vi "OperateClick.vi"(3 "XRef":refnum<vi>, 4 "Point":T1, 5 "State In":T3={"Input Type"=variant(dbl 0.0), "Width"=0, "Typedef Name"="", "Value Type"=variant, "Selection"=0, "Options"=[], "Selections"=[], "Display Selections"=[], "Element Names"=[], "Typedef Name Width"=0, "Display Selection Width"=[], "Code Generated"=FALSE}) -> (0 "Reply":string[](array[string]), 2 "State Out":T3={"Input Type"=variant(dbl 0.0), "Width"=0, "Typedef Name"="", "Value Type"=variant, "Selection"=0, "Options"=[], "Selections"=[], "Display Selections"=[], "Element Names"=[], "Typedef Name Width"=0, "Display Selection Width"=[], "Code Generated"=FALSE})   [LabVIEW 2015, in "Read-Write-Signals.xnode"]
doc: "This ability VI is called when a user operate clicks on your XNode. Point is the point of the click relative to the top-left corner of your XNode. If you wish to show a menu in response to a user's operate click, issue the reply \"ShowMenu\". It is an error to issue this reply if you have not implemented the BuildMenu and SelectMenu ability VIs.\n\nDefault behavior: None.\n\nThis ability provides UI and OS messages are handled.\n\nSee also: BuildMenu3, SelectMenu3"
uses:
  Read-Write-Signals.xnode
  State.ctl
  Read-Write-Signals Item.ctl
  Read-Write-Signals Sub Item.ctl
  Read-Write-Signals Sub Item Type.ctl
  Read-Write-Signals Selection.ctl
  Read-Write-Signals Display Selection.ctl
  <vilib>/XNodeSupport/XNodePoint.ctl
  <vilib>/XNodeSupport/XNodeInt.ctl
  <vilib>/XNodeSupport/NI_XNodeSupport.lvlib
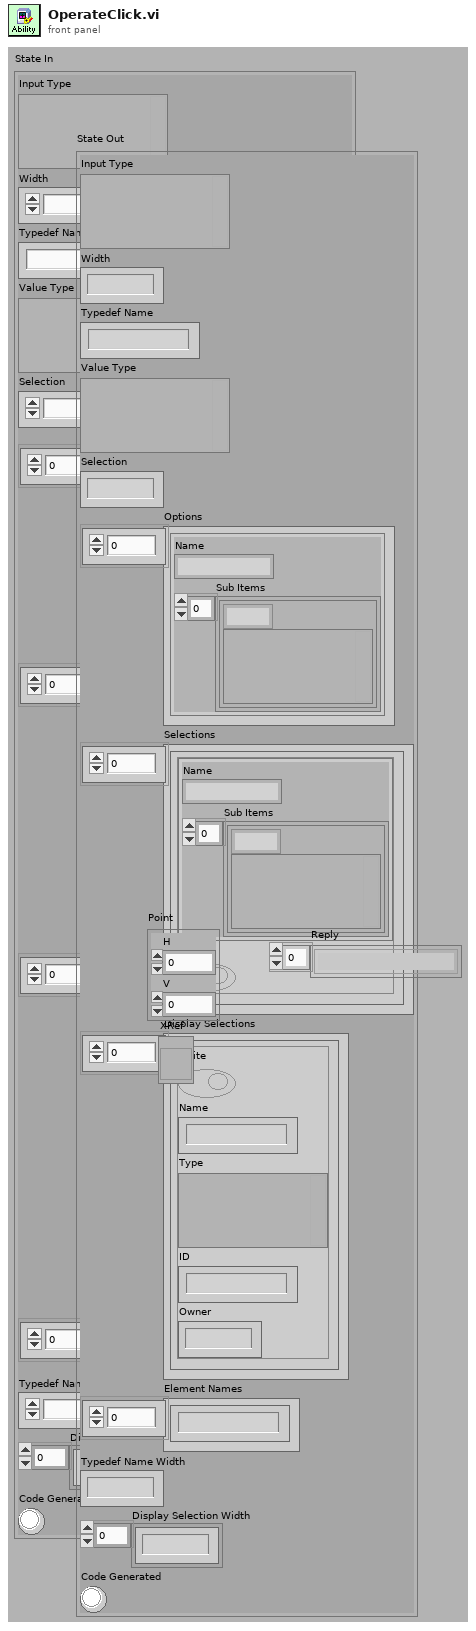
[diagram p1: front panel]
types:
  T1 = typedef "NI_XNodeSupport.lvlib/XNodePoint.ctl" = cluster{"H":T2, "V":T2}
  T2 = typedef "NI_XNodeSupport.lvlib/XNodeInt.ctl" = i32
  T3 = typedef "Read-Write-Signals.xnode/State.ctl" = cluster{"Input Type":variant, "Width":i32, "Typedef Name":string, "Value Type":variant, "Selection":i32, "Options":T4[], "Selections":T7[], "Display Selections":T8[], "Element Names":string[], "Typedef Name Width":i32, "Display Selection Width":i32[], "Code Generated":bool}
  T4 = typedef "Read-Write-Signals Item.ctl" = cluster{"Name":string, "Sub Items":T5[]}
  T5 = typedef "Read-Write-Signals Sub Item.ctl" = cluster{"Type":T6, "Value":variant}
  T6 = typedef "Read-Write-Signals Sub Item Type.ctl" = enum8{"Cluster Element", "Array Element", "Subarray"}
  T7 = typedef "Read-Write-Signals Selection.ctl" = cluster{"Item":T4, "Write":bool}
  T8 = typedef "Read-Write-Signals Display Selection.ctl" = cluster{"Write":bool, "Name":string, "Type":variant, "ID":string, "Owner":i32}
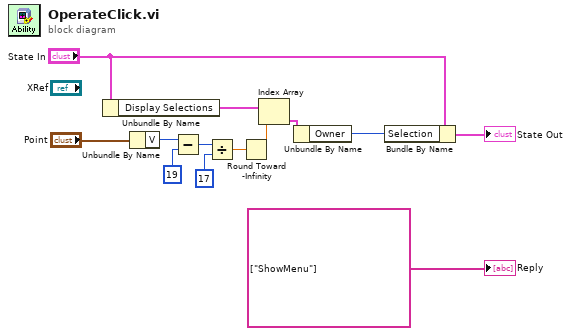
[diagram p0: block diagram]
diagram:
  n1 = Unbundle By Name("State In") -> ("Display Selections"=w5:T8[])
  n2 = Unbundle By Name("Point") -> ("V"=w10:T2)
  n3 = Subtract(x=w10, y=T2 19) -> (x-y=w13:T2)
  n4 = Divide(x=w13, y=T2 17) -> (x/y=w11:dbl)
  n5 = Round Toward -Infinity(1:w11) -> (0:w8:dbl)
  n6 = Index Array(array=w5, index=w8) -> (element=w6:T8)
  n7 = Unbundle By Name(w6) -> ("Owner"=w7:i32)
  n8 = Bundle By Name(cluster="State In", "Selection"=w7) -> (→"State Out":T3)
  "Reply" <- string[] ["ShowMenu"] ("Reply")
